vi "host_abortq.vi"() -> (0 "abort":bool)   [LabVIEW 2021]
doc: "Check if the scan is aborted or not."
uses:
  core/host_global_vars.vi
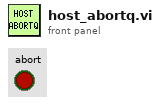
[diagram p1: front panel]
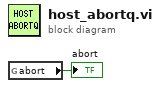
[diagram p0: block diagram]
diagram:
  n1 = global read "host_global_vars.vi" "abort"() -> (→"abort":bool)
